vi "Set Display Screen.vi"(8 "error in (no error)":errorcluster, 10 "Screen Home":u16(ring) items=["Home Screen", "Source Screen", "Plot Screen", "User-defined Screen", "Statistics Screen", "Settings Screen", "Graph Screen", "Data sheet Screen"], 11 "VISA resource name":refnum<visa-resource-name>) -> (0 "error out":errorcluster, 3 "VISA resource name out":refnum<visa-resource-name>)   [LabVIEW 2017, in "Keithley 2450.lvlib"]
doc: "This VI selects which front-panel screen is displayed.."
uses:
  Keithley 2450.lvlib
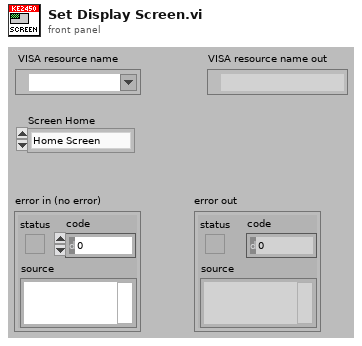
[diagram p1: front panel]
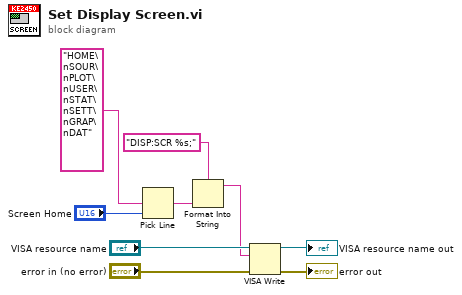
[diagram p0: block diagram]
diagram:
  n1 = Pick Line(multi-line string="HOME\nSOUR\nPLOT\nUSER\nSTAT\nSETT\nGRAP\nDAT", line index="Screen Home") -> (output string=w1:string)  [unwired: 1 in]
  n2 = Format Into String(format string="DISP:SCR %s;", w1) -> (resulting string=w4:string)  [unwired: 2 in, 1 out]
  n3 = VISA Write(VISA resource name="VISA resource name", write buffer=w4, error in (no error)="error in (no error)") -> (VISA resource name out=→"VISA resource name out":refnum<visa-resource-name>, error out=→"error out":errorcluster)  [unwired: 1 out]
